vi "Read Data Value.vi"(8 "error in (no error)":errorcluster, 10 "Data in":variant, 11 "DataReader in":refnum<class "DataReader.lvclass">) -> (0 "error out":errorcluster, 2 "Data out":variant, 3 "DataReader out":refnum<class "DataReader.lvclass">)   [LabVIEW 2020, in "Module.lvlib" / "DataReader.lvclass"]
uses:
  DataReader.lvclass
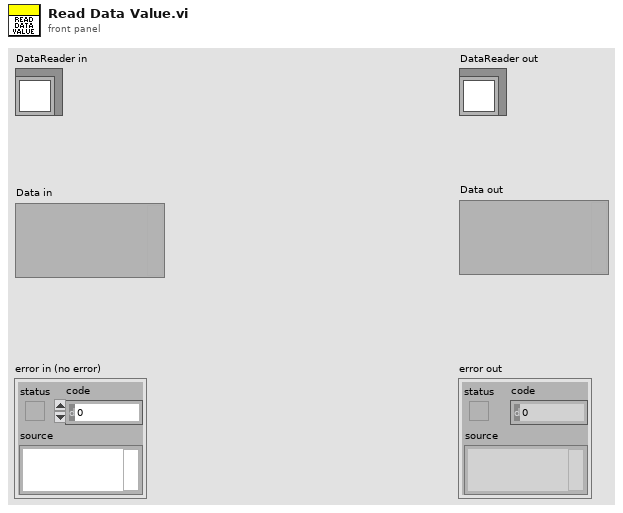
[diagram p1: front panel]
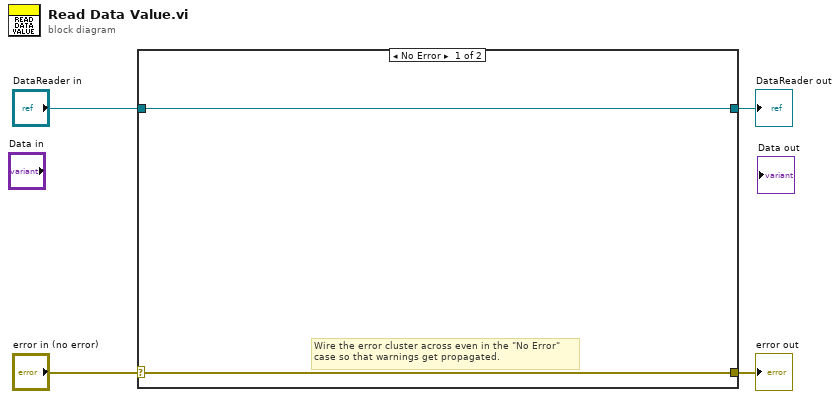
[diagram p0: block diagram]
diagram:
  n1 = case shown="No Error" "error in (no error)" {
    selector: "error in (no error)" -> [w5 w8]
    tunnel: [w5 w8] -> w3
    tunnel: [w6 w7] -> w1
    tunnel: "DataReader in" -> [w6 w7]
    frame No Error {
      # "Wire the error cluster across even in the \"No Error\"\ncase so that warnings get propagated."
    }
    frame Error {
    }
  }
  "error out" <- w3
  "DataReader out" <- w1
